vi "Simple_Inverse.vi"(8 "L 2":dbl(slide)=75.0 scale=0.0..200.0, 9 "L 1":dbl(slide)=75.0 scale=0.0..200.0, 11 "end effector":cluster{dbl, dbl}={5.662, 105.69} {"?" format="%.1f"; "?" format="%#.1f"}) -> (0 "Angle 2":dbl(knob)=-90.24225061853012 scale=-90.0..90.0, 1 "Angle1":dbl(knob)=42.054620502414885 scale=-90.0..90.0)   [LabVIEW 2024]
panel:
  out "2D Picture":picture
  # "mm"
  # "mm"
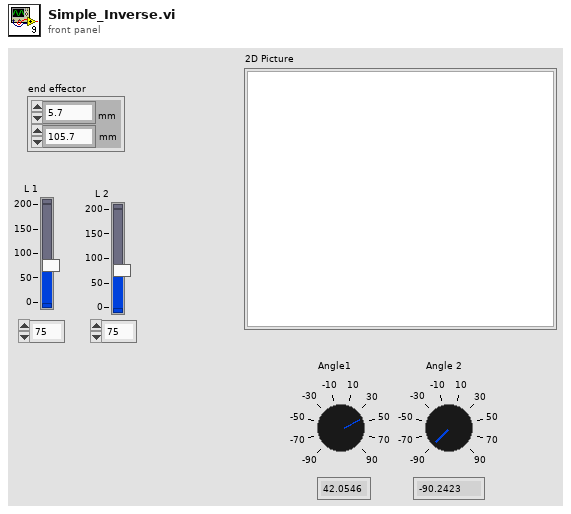
[diagram p1: front panel]
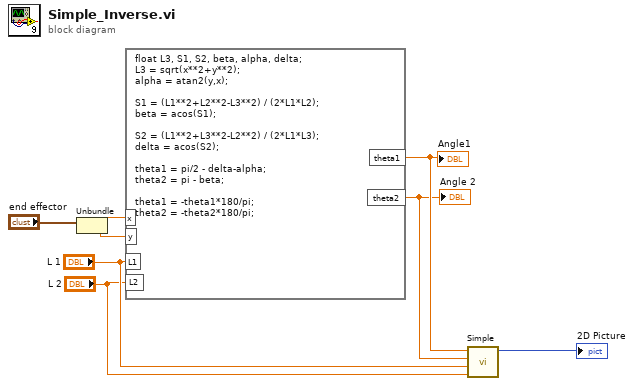
[diagram p0: block diagram]
diagram:
  n1 = Unbundle("end effector") -> (w7:dbl, w6:dbl)
  n2 = formula code="float L3, S1, S2, beta, alpha, delta;\nL3 = sqrt(x**2+y**2);\nalpha = atan2(y,x);\n\nS1 = (L1**2+L2**2-L3**2) / (2*L1*L2);\nbeta = acos(S1);\n\nS2 = (L1**2+L3**2-L2**2) / (2*L1*L3);\ndelta = acos(S2);\n\ntheta1 = pi/2 - delta-alpha;\ntheta2 = pi - beta;\n\ntheta1 = -theta1*180/pi;\ntheta2 = -theta2*180/pi;"("L1"="L 1", "L2"="L 2", "x"=w7, "y"=w6) -> ("theta1"=w4:dbl, "theta2"=w3:dbl)
  "Angle1" <- w4
  "Angle 2" <- w3
  n3 = call "Simple.vi"("L 2"="L 2", "L 1"="L 1", "Angle 2"=w3, "Angle1"=w4) -> ("2D Picture"=→"2D Picture":picture)  [unwired: 5 in, 2 out]
